vi "ramp (1 sec).vi"(6 "gain":dbl=1.0, 8 "TeleOp Elapsed Seconds":dbl, 11 "target":dbl format="%#_13g") -> (3 "output":dbl format="%#_13g")   [LabVIEW 2014]
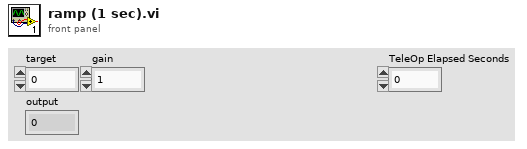
[diagram p1: front panel]
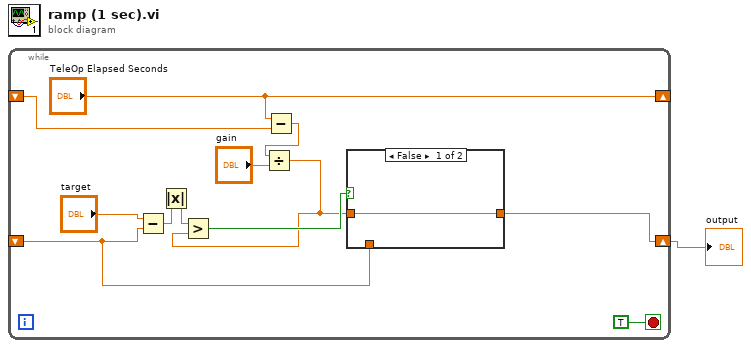
[diagram p0: block diagram]
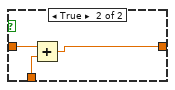
[diagram p2: hidden frame]
diagram:
  n1 = while {
    shift-right: ["TeleOp Elapsed Seconds"] -> _
    shift-left: _ -> [w12]
    shift-right: [w9] -> w1
    shift-left: _ -> [w6]
    stop <- TRUE stop-if-true
    n2 = Subtract(x="target", y=w6) -> (x-y=w8:dbl)
    n3 = Absolute Value(x=w8) -> (abs(x)=w7:dbl)
    n4 = Subtract(x="TeleOp Elapsed Seconds", y=w12) -> (x-y=w4:dbl)
    n5 = Divide(x=w4, y="gain") -> (x/y=w3:dbl)
    n6 = Greater?(x=w7, y=w3) -> (0:w10:bool)
    n7 = case shown="False" w10 {
      tunnel: w3 -> [w14 w17]
      tunnel: [w14 w15] -> w9
      tunnel: w6 -> [_ w16]
      frame False {
      }
      frame True {
        n8 = Add(x=w17, y=w16) -> (x+y=w15:dbl)
      }
    }
  }
  "output" <- w1
